vi "Harsha's Dumb Disgusting Auto Engage.vi"(0 "State":T1, 1 "Operation":T12, 2 "Roll":dbl, 5 "Boolean in":bool, 7 "Pitch":dbl, 9 "Motors":T2 {"Radii (ft)"."Right Back Position" format="%.2f"; "Radii (ft)"."Right Front Position" format="%.2f"; "Radii (ft)"."Left Back Position" format="%.2f"; "Radii (ft)"."Left Front Position" format="%.2f"; "Pigeon2"."Type" items=["CAN"=352321536, "TalonSRX"=33554432]}, 12 "Cluster":cluster{"Start Time (ms)":u32, "Iterations":i32}, 13 "millisecond timer value":u32, 14 "Heading":bool) -> (3 "Waveform Chart":cluster{"Yaw":dbl, "Pitch":dbl, "Roll":dbl}(graph), 4 "Boolean 3":bool, 6 "Waveform Chart 2":T13(graph), 8 "Boolean out":bool, 10 "Infinite":dbl, 15 "New State":T1)   [LabVIEW 2020]
uses:
  Angle State.ctl
  Drive Operations.ctl
  swerve/Type Definitions/Hardware/Swerve Drives/(NEO-NEO-ThroughBore-Pigeon2) Swerve.ctl
  swerve/Type Definitions/Hardware/4 Motor Sets/(NEO & NEO 550) 4 Motor Set.ctl
  <vilib>/Rock Robotics/WPI/MotorControl/WPI_MotorControlDeviceRef.ctl
  <vilib>/Rock Robotics/WPI/MotorControl/WPI_MotorControlType.ctl
  <vilib>/Rock Robotics/SystemInterfaces/DIO/FPGA_DIOPWMChannel.ctl
  <vilib>/Rock Robotics/WPI/PWM/WPI_PWMDeadband.ctl
  <vilib>/Rock Robotics/SystemInterfaces/DIO/FPGA_DIOChannel.ctl
  <vilib>/Rock Robotics/WPI/ThirdParty/Phoenix-LabVIEW/Pigeon IMU/CTRE_PigeonIMU_DeviceRef.ctl
  <vilib>/Rock Robotics/WPI/ThirdParty/Phoenix-LabVIEW/Pigeon IMU/CTRE_PigeonIMU_ConnectionType.ctl
  swerve/Type Definitions/Data/Pod Positions.ctl
  swerve/Type Definitions/Data/Robot Velocities.ctl
  <vilib>/Rock Robotics/WPI/ThirdParty/Phoenix-LabVIEW/Pigeon IMU/CTRE_PigeonIMU_GetYPR.vi
  <vilib>/Rock Robotics/Network Tables/NT Read Boolean.vi
  <vilib>/Rock Robotics/Network Tables/NT Read Number.vi
  <vilib>/ptbypt/NI_PtbyPt.lvlib
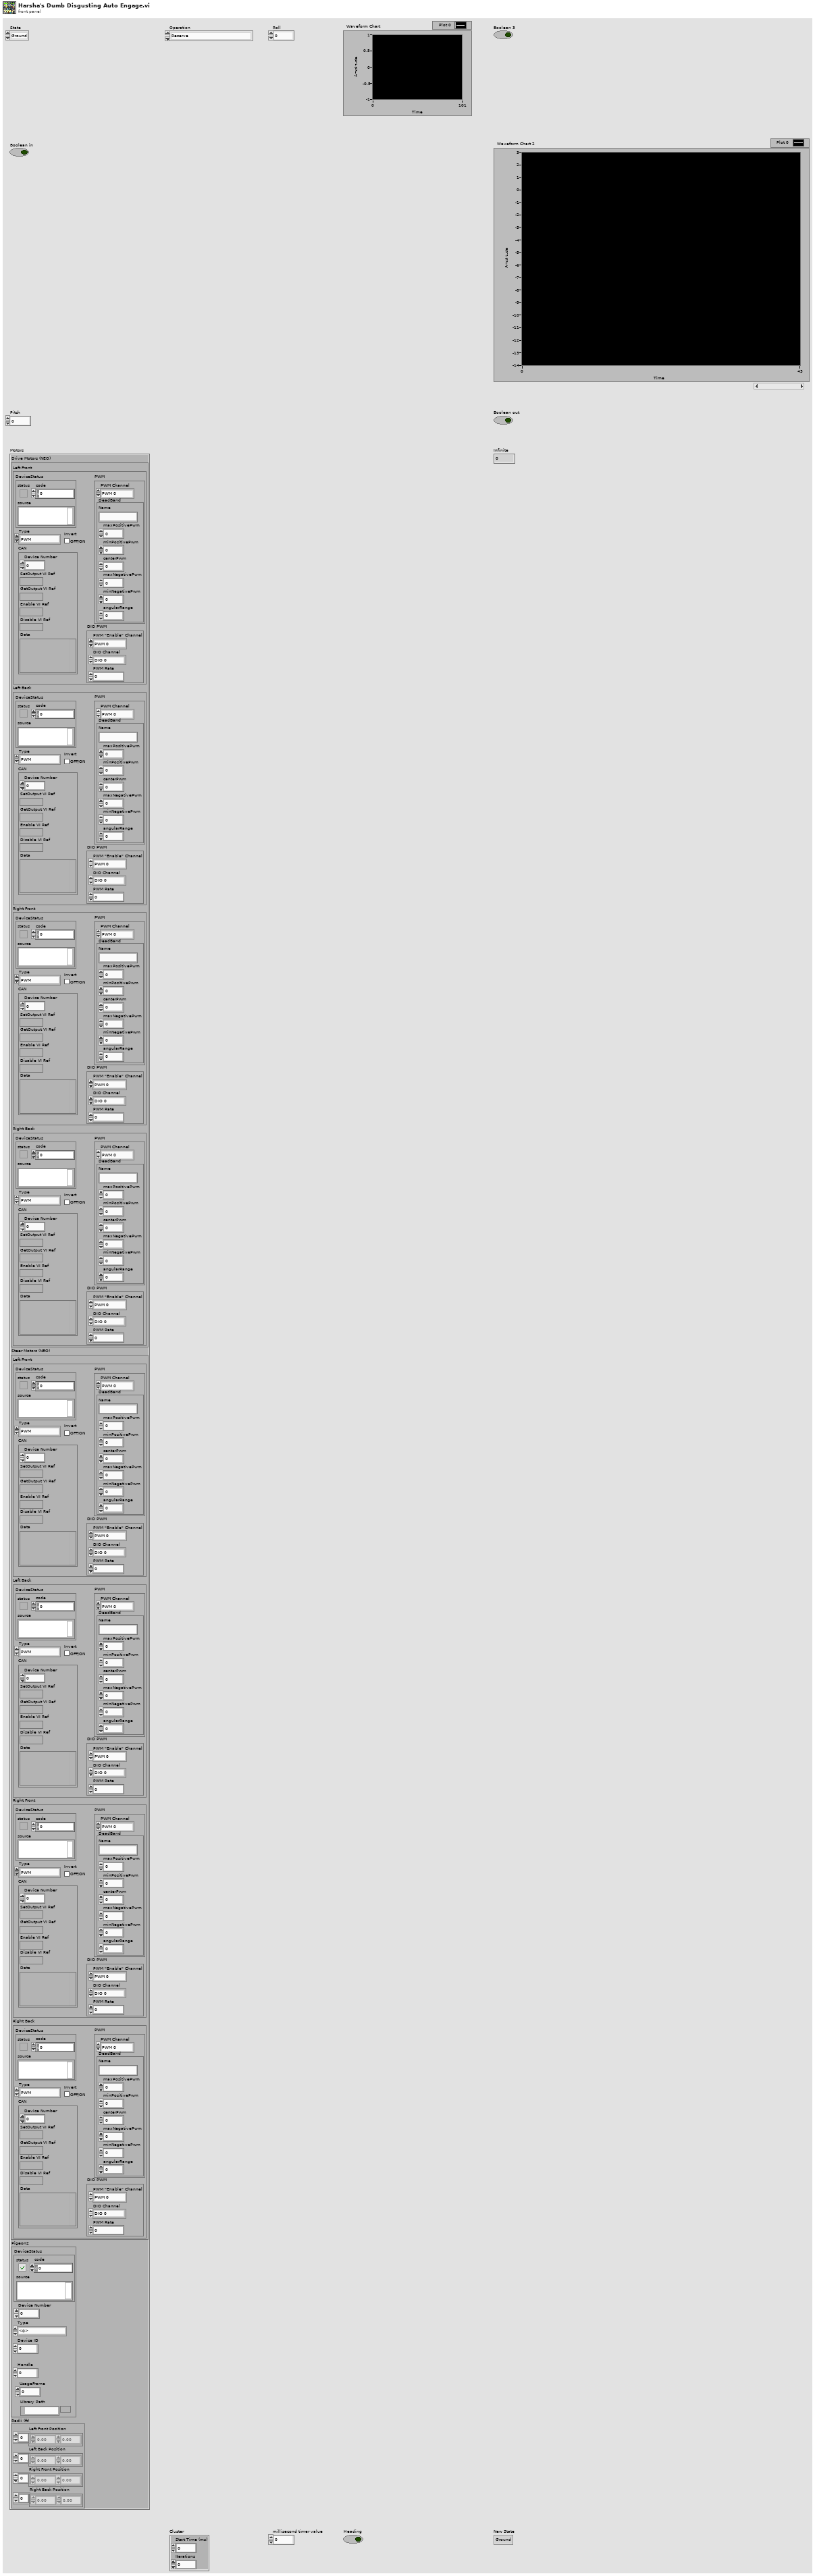
[diagram p1: front panel]
types:
  T1 = typedef "Angle State.ctl" = enum16{"Ground", "Close to balanced", "Balanced", "Tilted"}
  T2 = typedef "(NEO-NEO-ThroughBore-Pigeon2) Swerve.ctl" = cluster{"Drive Motors (NEO)":T3, "Steer Motors (NEO)":T3, "Pigeon2":T9, "Radii (ft)":T11}
  T3 = typedef "(NEO & NEO 550) 4 Motor Set.ctl" = cluster{"Left Front":T4, "Left Back":T4, "Right Front":T4, "Right Back":T4}
  T4 = typedef "WPI_MotorControlDeviceRef.ctl" = cluster{"DeviceStatus":errorcluster, "Type":T5, "PWM":cluster{"PWM Channel":T6, "DeadBand":T7}, "CAN":cluster{"Device Number":u8, "SetOutput VI Ref":variant, "GetOutput VI Ref":variant, "Enable VI Ref":variant, "Disable VI Ref":variant, "Data":variant}, "Invert":bool, "DIO PWM":cluster{"PWM \"Enable\" Channel":T6, "DIOChannel":T8, "PWM Rate":dbl}}
  T5 = typedef "WPI_MotorControlType.ctl" = enum16{"PWM", "CAN", "DIO PWM"}
  T6 = typedef "FPGA_DIOPWMChannel.ctl" = enum8{"PWM 0", "PWM 1", "PWM 2", "PWM 3", "PWM 4", "PWM 5", "PWM 6", "PWM 7", "PWM 8", "PWM 9", "PWM MXP 0", "PWM MXP 1", "PWM MXP 2", "PWM MXP 3", "PWM MXP 4", "PWM MXP 5", "PWM MXP 6", "PWM MXP 7", "PWM MXP 8", "PWM MXP 9", "Invalid"}
  T7 = typedef "WPI_PWMDeadband.ctl" = cluster{"Name":string, "maxPositivePwm":i32, "minPositivePwm":i32, "centerPwm":i32, "maxNegativePwm":i32, "minNegativePwm":i32, "angularRange":u16}
  T8 = typedef "FPGA_DIOChannel.ctl" = enum8{"DIO 0", "DIO 1", "DIO 2", "DIO 3", "DIO 4", "DIO 5", "DIO 6", "DIO 7", "DIO 8", "DIO 9", "DIO MXP 0", "DIO MXP 1", "DIO MXP 2", "DIO MXP 3", "DIO MXP 4", "DIO MXP 5", "DIO MXP 6", "DIO MXP 7", "DIO MXP 8", "DIO MXP 9", "DIO MXP 10", "DIO MXP 11", "DIO MXP 12", "DIO MXP 13", "DIO MXP 14", "DIO MXP 15", "SPI Port CS1", "SPI Port CS2", "SPI Port CS3", "SPI Port MISO", "SPI Port MOSI", "Invalid"}
  T9 = typedef "CTRE_PigeonIMU_DeviceRef.ctl" = cluster{"DeviceStatus":errorcluster, "Device Number":u8, "Type":T10, "Device ID":u32, "Handle":u64, "UsageFrame":u32, "Library Path":path}
  T10 = typedef "CTRE_PigeonIMU_ConnectionType.ctl" = u32
  T11 = typedef "Pod Positions.ctl" = cluster{"Left Front Position":dbl[], "Left Back Position":dbl[], "Right Front Position":dbl[], "Right Back Position":dbl[]}
  T12 = typedef "Drive Operations.ctl" = enum16{"Reserve", "Read Current", "Immediate", "Calibrate", "Auto", "Auto Engage", "Brake"}
  T13 = cluster{"standard deviation":dbl, "mean":dbl, dbl}
  T14 = cluster{"Field Centric?":bool, "SnapToScore":bool, "TranslationalAlign":bool}
  T15 = typedef "Robot Velocities.ctl" = cluster{"X Velocity":dbl, "Y Velocity":dbl, "Rotational \nVelocity":dbl}
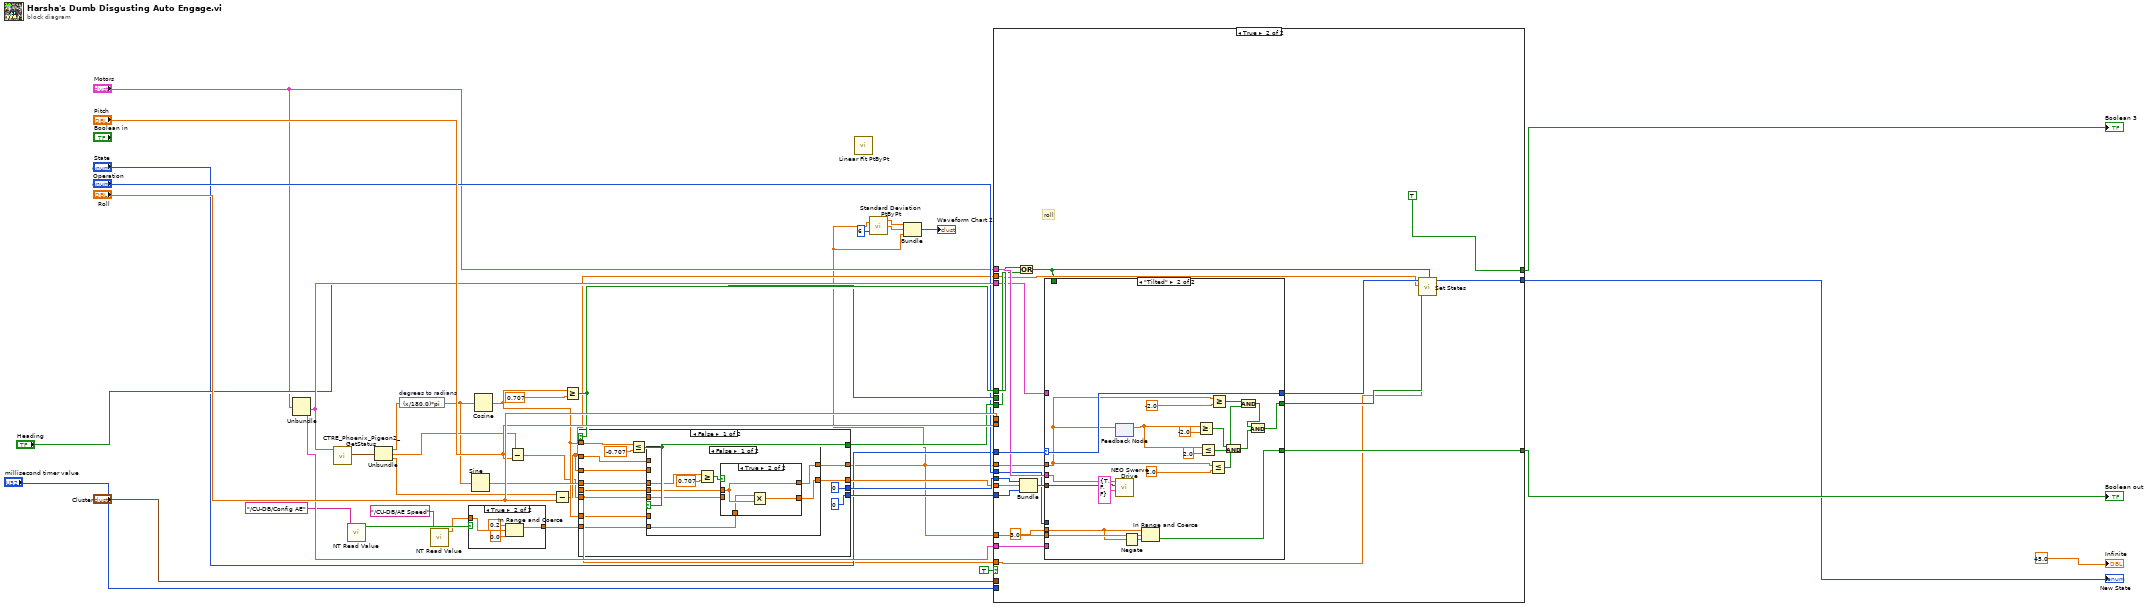
[diagram p0: block diagram]
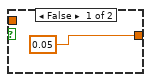
[diagram p2: hidden frame]
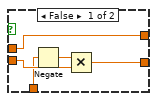
[diagram p3: hidden frame]
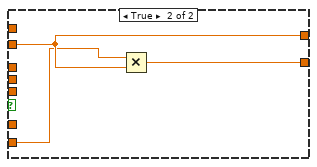
[diagram p4: hidden frame]
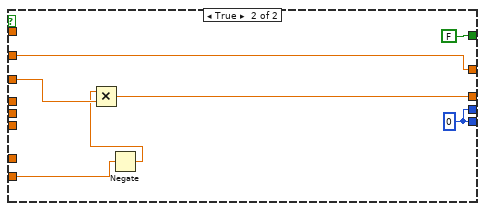
[diagram p5: hidden frame]
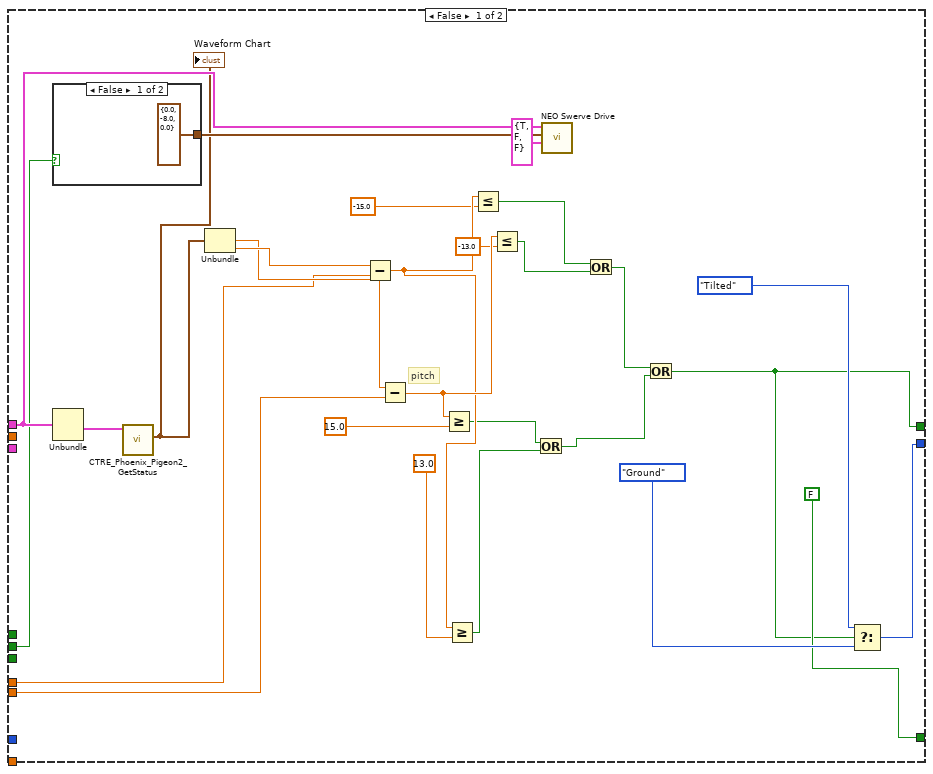
[diagram p6: hidden frame]
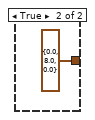
[diagram p7: hidden frame]
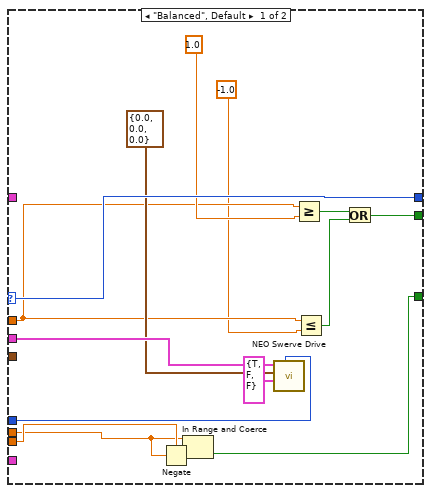
[diagram p8: hidden frame]
diagram:
  n1 = Unbundle("Motors") -> ("Pigeon2"=w33:T9, "Radii (ft)"=w32:T11)  [unwired: 2 out]
  n2 = call-poly <vilib>:"CTRE_Phoenix_Pigeon2_GetStatus.vi"("PigeonIMUDevRef"=w33) -> ("Yaw Pitch Roll"=w26:cluster{"Yaw":dbl, "Pitch":dbl, "Roll":dbl})  [unwired: 8 in, 2 out]
  n3 = call-poly <vilib>:"NT Read Value.vi"("name"="/CU-DB/Config AE") -> ("value"=w5:bool)  [unwired: 8 in, 2 out]
  n4 = Unbundle(w26) -> ("Yaw"=w21:dbl, "Pitch"=w22:dbl, "Roll"=w23:dbl)
  n5 = expression code="(x/180.0)*pi" "degrees to radians"(w21) -> (w20:dbl)
  n6 = call-poly <vilib>:"NT Read Value.vi"("name"="/CU-DB/AE Speed") -> ("value"=w4:dbl)  [unwired: 8 in, 2 out]
  n7 = case shown="True" w5 {
    tunnel: [0.05 w45] -> w6
    tunnel: w4 -> [_ w44]
    frame False {
    }
    frame True {
      n8 = In Range and Coerce(upper limit=0.2, x=w44, lower limit=0.0) -> (coerced(x)=w45:dbl)  [unwired: 1 out]
    }
  }
  n9 = Sine(x=w20) -> (sin(x)=w25:dbl)
  n10 = Cosine(x=w20) -> (cos(x)=w24:dbl)
  n11 = Subtract(x=w22, y="Pitch") -> (x-y=w7:dbl)
  n12 = Subtract(x=w23, y="Roll") -> (x-y=w8:dbl)
  n13 = Greater Or Equal?(x=w24, y=0.707) -> (x >= y?=w28:bool)
  n14 = case shown="False" w28 {
    tunnel: w8 -> [w47 w82]
    tunnel: w25 -> [w53 _]
    tunnel: w24 -> [w58 _]
    tunnel: w7 -> [w55 _]
    tunnel: [w52 w83] -> w29
    tunnel: [0 w85] -> w34
    tunnel: [0 w85] -> w30
    tunnel: w24 -> [w54 _]
    tunnel: [w50 w84] -> w1
    tunnel: w8 -> [w51 w84]
    tunnel: w7 -> [w49 _]
    tunnel: [w48 FALSE] -> w31
    tunnel: w6 -> [w46 w80]
    frame False {
      n15 = Less Or Equal?(x=w54, y=-0.707) -> (x <= y?=w48:bool)
      n16 = case shown="False" w48 {
        tunnel: w55 -> [w64 _]
        tunnel: [w63 w78] -> w52
        tunnel: w58 -> [_ _]
        tunnel: w53 -> [w65 _]
        tunnel: [w61 w77] -> w50
        tunnel: w51 -> [_ _]
        tunnel: w49 -> [w62 _]
        tunnel: w47 -> [_ w77]
        tunnel: w46 -> [w60 w76]
        frame False {
          n17 = Greater Or Equal?(x=w65, y=0.707) -> (x >= y?=w66:bool)
          n18 = case shown="True" w66 {
            tunnel: [w70 w74] -> w63
            tunnel: w64 -> [w71 _]
            tunnel: w62 -> [w72 w75]
            tunnel: [w72 w75] -> w61
            tunnel: w60 -> [w69 w73]
            frame False {
              n19 = Negate(x=w69) -> (-x=w68:dbl)
              n20 = Multiply(x=w68, y=w71) -> (x*y=w70:dbl)
            }
            frame True {
              n21 = Multiply(x=w73, y=w75) -> (x*y=w74:dbl)
            }
          }
        }
        frame True {
          n22 = Multiply(x=w76, y=w77) -> (x*y=w78:dbl)
        }
      }
    }
    frame True {
      w85 = 0
      n23 = Negate(x=w80) -> (-x=w79:dbl)
      n24 = Multiply(x=w79, y=w82) -> (x*y=w83:dbl)
    }
  }
  n25 = call <vilib>:"Linear Fit PtByPt.vi"() -> ()  [unwired: 11 in, 5 out]
  n26 = call <vilib>:"Standard Deviation PtByPt.vi"("x"=w1, "sample length"=6) -> ("standard deviation"=w36:dbl, "mean"=w37:dbl)  [unwired: 1 in, 1 out]
  n27 = Bundle("standard deviation"=w36, "mean"=w37, w1) -> (→"Waveform Chart 2":T13)  [unwired: 1 in]
  n28 = case shown="True" TRUE {
    tunnel: "State" -> [_ w136]
    tunnel: "Motors" -> [w109 w135]
    tunnel: "Operation" -> [_ w133]
    tunnel: "Cluster" -> [_ _]
    tunnel: "millisecond timer value" -> [_ _]
    tunnel: [w105 w130] -> w16
    tunnel: "Heading" -> [w108 _]
    tunnel: [w92 TRUE] -> w18
    tunnel: [FALSE w128] -> w19
    tunnel: w7 -> [_ w127]
    tunnel: w28 -> [_ w126]
    tunnel: w29 -> [_ w125]
    tunnel: w34 -> [_ w124]
    tunnel: w30 -> [_ w123]
    tunnel: w1 -> [_ w118]
    tunnel: w31 -> [_ w122]
    tunnel: w8 -> [_ w121]
    tunnel: w33 -> [_ w120]
    tunnel: w32 -> [_ w119]
    tunnel: "Pitch" -> [w88 _]
    tunnel: "Roll" -> [w87 _]
    tunnel: w1 -> [_ w116]
    frame False {
      # "pitch"
      n29 = case shown="False" w108 {
        tunnel: [T15 {"X Velocity"=0.0, "Y Velocity"=-8.0, "Rotational \nVelocity"=0.0} ("Robot Velocities") T15 {"X Velocity"=0.0, "Y Velocity"=8.0, "Rotational \nVelocity"=0.0} ("Robot Velocities")] -> w112
        frame False {
        }
        frame True {
        }
      }
      n30 = Unbundle(w109) -> ("Pigeon2"=w111:T9)  [unwired: 3 out]
      n31 = call-poly <vilib>:"CTRE_Phoenix_Pigeon2_GetStatus.vi"("PigeonIMUDevRef"=w111) -> ("Yaw Pitch Roll"=w103:cluster{"Yaw":dbl, "Pitch":dbl, "Roll":dbl})  [unwired: 8 in, 2 out]
      "Waveform Chart" <- w103
      n32 = Unbundle(w103) -> ("Pitch"=w102:dbl, "Roll"=w110:dbl)  [unwired: 1 out]
      n33 = Subtract(x=w110, y=w87) -> (x-y=w99:dbl)
      n34 = Subtract(x=w102, y=w88) -> (x-y=w101:dbl)
      n35 = Greater Or Equal?(x=w101, y=15.0) -> (x >= y?=w96:bool)
      n36 = Greater Or Equal?(x=w99, y=13.0) -> (x >= y?=w95:bool)
      n37 = Less Or Equal?(x=w99, y=-15.0) -> (x <= y?=w98:bool)
      n38 = Less Or Equal?(x=w101, y=-13.0) -> (x <= y?=w97:bool)
      n39 = Or(x=w96, y=w95) -> (x .or. y?=w93:bool)
      n40 = call "NEO Swerve Drive.vi"("Drive Conditions"=T14 {"Field Centric?"=TRUE, "SnapToScore"=FALSE, "TranslationalAlign"=FALSE}, "Robot Velocities"=w112, "Swerve Drive"=w109) -> ()  [unwired: 8 in, 1 out]
      n41 = Or(x=w98, y=w97) -> (x .or. y?=w94:bool)
      n42 = Or(x=w94, y=w93) -> (x .or. y?=w92:bool)
      n43 = Select(t=Angle_State."Tilted" ("State 2"), s=w92, f=Angle_State."Ground" ("State 2")) -> (s? t:f=w105:T1)
    }
    frame True {
      # "roll"
      n44 = Or(x=w126, y=w122) -> (x .or. y?=w117:bool)
      n45 = Bundle(w123, w125, w124) -> (w134:cluster{i32, dbl, i32})  [unwired: 1 in]
      n46 = case shown="\"Tilted\"" w136 {
        selector: w136 -> [w151 w170]
        tunnel: w120 -> [_ _]
        tunnel: w119 -> [_ _]
        tunnel: w135 -> [w150 w169]
        tunnel: w134 -> [_ w168]
        tunnel: w133 -> [w142 _]
        tunnel: w118 -> [w145 w165]
        tunnel: [w151 w170] -> w131
        tunnel: [w143 w157] -> w132
        tunnel: [w139 w154] -> w128
        tunnel: w117 -> [_ _]
        tunnel: w116 -> [w140 w155]
        tunnel: 3.0 ("upper limit") -> [w138 w153]
        frame "Balanced", Default {
          n47 = Negate(x=w138) -> (-x=w137:dbl)
          n48 = In Range and Coerce(upper limit=w138, x=w140, lower limit=w137) -> (In Range?=w139:bool)  [unwired: 1 out]
          n49 = call "NEO Swerve Drive.vi"("Operation"=w142, "Drive Conditions"=T14 {"Field Centric?"=TRUE, "SnapToScore"=FALSE, "TranslationalAlign"=FALSE}, "Robot Velocities"=T15 {"X Velocity"=0.0, "Y Velocity"=0.0, "Rotational \nVelocity"=0.0}, "Swerve Drive"=w150) -> ()  [unwired: 7 in, 1 out]
          n50 = Greater Or Equal?(x=w145, y=1.0) -> (x >= y?=w148:bool)
          n51 = Less Or Equal?(x=w145, y=-1.0) -> (x <= y?=w147:bool)
          n52 = Or(x=w148, y=w147) -> (x .or. y?=w143:bool)
        }
        frame "Tilted" {
          n53 = feedback-in #1(w165) -> ()
          n54 = feedback #1() -> (w163:dbl)  [unwired: 1 in]
          n55 = call "NEO Swerve Drive.vi"("Drive Conditions"=T14 {"Field Centric?"=TRUE, "SnapToScore"=FALSE, "TranslationalAlign"=FALSE}, "Robot Velocities"=w168, "Swerve Drive"=w169) -> ()  [unwired: 8 in, 1 out]
          n56 = Negate(x=w153) -> (-x=w152:dbl)
          n57 = In Range and Coerce(upper limit=w153, x=w155, lower limit=w152) -> (In Range?=w154:bool)  [unwired: 1 out]
          n58 = Greater Or Equal?(x=w163, y=-2.0) -> (x >= y?=w160:bool)
          n59 = Less Or Equal?(x=w163, y=2.0) -> (x <= y?=w161:bool)
          n60 = Less Or Equal?(x=w165, y=2.0) -> (x <= y?=w166:bool)
          n61 = Greater Or Equal?(x=w165, y=-2.0) -> (x >= y?=w167:bool)
          n62 = And(x=w160, y=w161) -> (x .and. y?=w158:bool)
          n63 = And(x=w167, y=w166) -> (x .and. y?=w159:bool)
          n64 = And(x=w159, y=w158) -> (x .and. y?=w157:bool)
        }
      }
      n65 = call "Set States.vi"("Pitch?"=w117, "Roll"=w127, "Change State"=w132, "Pitch"=w121, "State"=w131) -> ("New State"=w130:T1)  [unwired: 6 in]
    }
  }
  "Boolean out" <- w19
  "Boolean 3" <- w18
  "New State" <- w16
  "Infinite" <- 45.0 ("Infinite")
